vi "Process Column Width.vi"(8 "Column":i32, 9 "Width":u32, 10 "error in (no error)":errorcluster) -> (1 "Stop?":bool, 2 "error out":errorcluster, 3 "Col Width[]":u32[](array[numeric]))   [LabVIEW 2020, in "Save Restore Settings.lvclass"]
uses:
  <userlib>/_MGI/Application Control/MGI Save Restore Settings/Save Restore Settings.lvclass
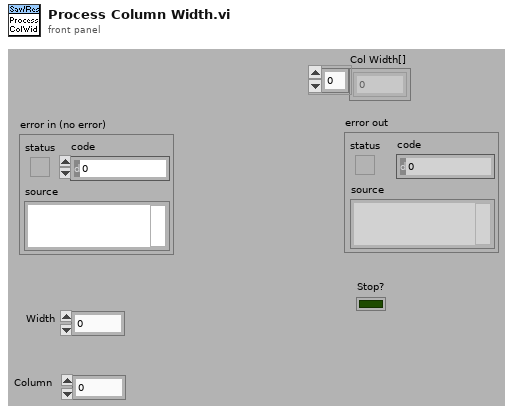
[diagram p1: front panel]
types:
  T1 = cluster{"Default":u32, "#Consec Defaults":i32, "Width[]":i32[]}
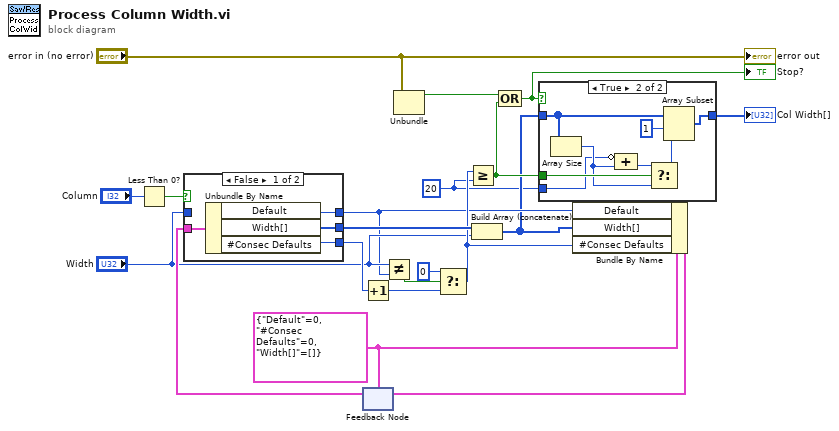
[diagram p0: block diagram]
diagram:
  w3 = 20 ("y")
  w10 = T1 {"Default"=0, "#Consec Defaults"=0, "Width[]"=[]} ("cluster")
  n1 = Less Than 0?(x="Column") -> (x < 0?=w1:bool)
  n2 = feedback #1(w10) -> (w17:T1)
  n3 = case shown="False" w1 {
    tunnel: w17 -> [w24 _]
    tunnel: [w23 _] -> w16
    tunnel: [w22 _] -> w11
    tunnel: [w21 w25] -> w5
    tunnel: "Width" -> [_ w25]
    frame False {
      n4 = Unbundle By Name(w24) -> ("Default"=w21:u32, "Width[]"=w22:i32[], "#Consec Defaults"=w23:i32)
    }
    frame True {
    }
  }
  n5 = Increment(x=w16) -> (x+1=w14:i32)
  n6 = Not Equal?(x="Width", y=w5) -> (x != y?=w13:bool)
  n7 = Unbundle("error in (no error)") -> ("status"=w15:bool)  [unwired: 2 out]
  n8 = Select(t=0, s=w13, f=w14) -> (s? t:f=w9:i32)
  n9 = Greater Or Equal?(x=w9, y=w3) -> (x >= y?=w20:bool)
  n10 = Build Array (concatenate)(w11, "Width") -> (w4:u32[])
  n11 = Compound Arithmetic op=OR(w15, w20) -> (w7:bool)
  "Stop?" <- w7
  n12 = case shown="True" w7 {
    tunnel: w20 -> [_ w32]
    tunnel: [_ w29] -> w18
    tunnel: w4 -> [_ w27]
    tunnel: w3 -> [_ w26]
    frame False {
    }
    frame True {
      n13 = Array Size(array=w27) -> (size(s)=w28:i32)
      n14 = Compound Arithmetic op=ADD(invert w26, w28) -> (w31:i32)
      n15 = Select(t=w31, s=w32, f=w28) -> (s? t:f=w30:i32)
      n16 = Array Subset(array=w27, index=1, length=w30) -> (w29:u32[])
    }
  }
  "Col Width[]" <- w18
  n17 = Bundle By Name(cluster=w10, "Default"=w5, "Width[]"=w4, "#Consec Defaults"=w9) -> (w8:T1)
  n18 = feedback-in #1(w8) -> ()
  "error out" <- "error in (no error)"
